vi "flat secuence local.vi"() -> ()   [LabVIEW 2020]
panel:
  out "Boolean":bool
  out "Meter":dbl(knob) scale=0.0..20.0
  in  "Motor2":dbl(knob) scale=0.0..10.0
  in  "Moto1":dbl(knob) scale=0.0..10.0
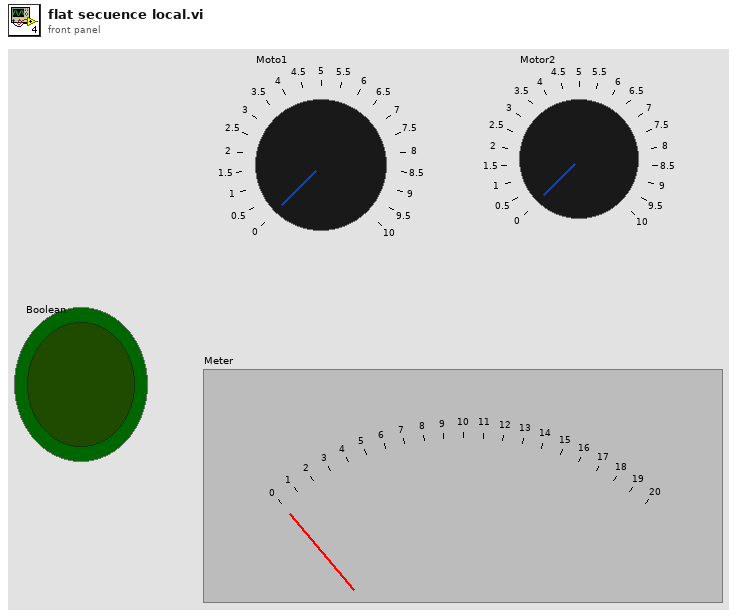
[diagram p1: front panel]
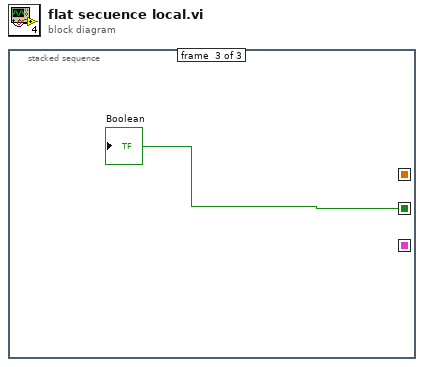
[diagram p0: block diagram]
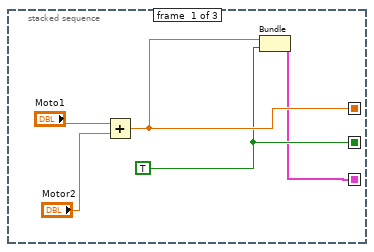
[diagram p2: hidden frame]
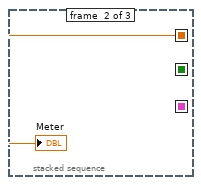
[diagram p3: hidden frame]
diagram:
  n1 = stacked-sequence {
    seq-local: [w3 _ _] -> [_ w6 _]
    seq-local: [w2 _ _] -> [_ _ w7]
    seq-local: [w1 _ _] -> [_ _ _]
    frame #0 {
      w2 = TRUE
      n2 = Add(x="Moto1", y="Motor2") -> (x+y=w3:dbl)
      n3 = Bundle(w3, w2) -> (w1:cluster{dbl, bool})  [unwired: 1 in]
    }
    frame #1 {
      "Meter" <- w6
    }
    frame #2 {
      "Boolean" <- w7
    }
  }
